vi "factory Reset.vi"(7 "option":u8, 8 "error in (no error)":errorcluster, 9 "id":u8, 10 "protocol_version":i32, 11 "port_num":i32) -> (0 "error out":errorcluster)   [LabVIEW 2018, in "labview.lvlib"]
doc: "WINDECLSPEC void factoryReset (int port_num, int protocol_version, uint8_t id, uint8_t option);"
uses:
  labview.lvlib
  dxl_x86_c.dll
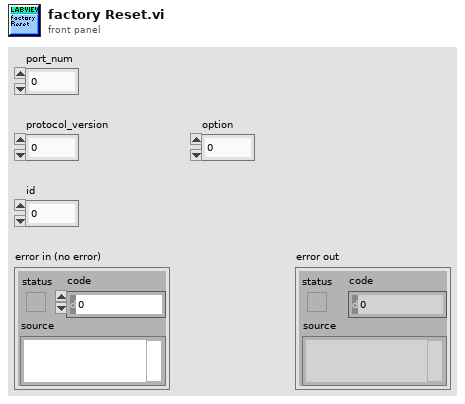
[diagram p1: front panel]
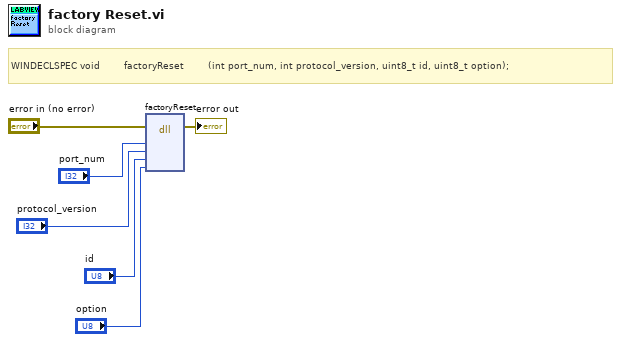
[diagram p0: block diagram]
diagram:
  # "WINDECLSPEC void        factoryReset        (int port_num, int protocol_version, uint8_t id, uint8_t option);"
  n1 = dll-call lib="C:/Users/joaos/OneDrive/Documents/[PhD]/Project Omnidirectional Vehicle/Vanes/LabView_code/joaoandthethreestands/DynamixelSDK-3.7.31/labview/new_compilation/dxl_x86_c.*" fn="factoryReset"(error in="error in (no error)", "port_num"="port_num", "protocol_version"="protocol_version", "id"="id", "option"="option") -> (error out=→"error out":errorcluster)  [unwired: 7 in, 1 out]
